vi "胜负对话.vi"(0 "黑子胜？":bool, 1 "白子胜？":bool, 6 "行或列":dbl) -> (14 "x .or. y?":bool, 19 "退出循环？":bool)   [LabVIEW 2018]
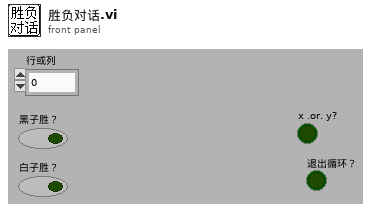
[diagram p1: front panel]
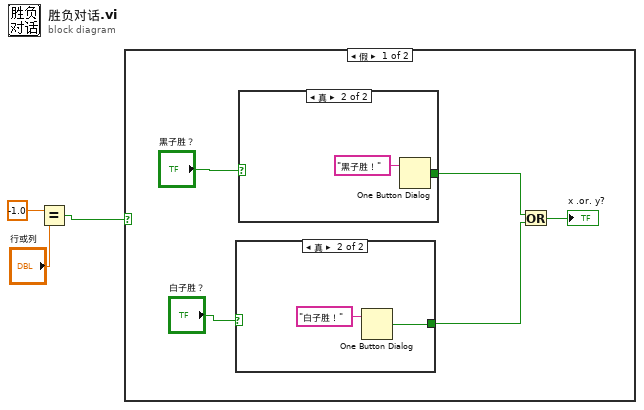
[diagram p0: block diagram]
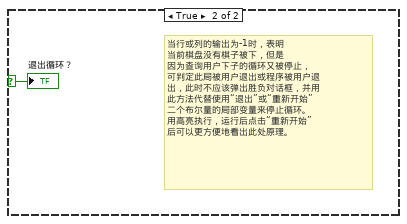
[diagram p4: hidden frame]
diagram:
  n1 = Equal?(x=-1.0, y="行或列") -> (x = y?=w3:bool)
  n2 = case shown="假" w3 {
    selector: w3 -> [_ w13]
    frame False {
      n3 = case shown="真" "白子胜？" {
        tunnel: [_ w9] -> w5
        frame False {
        }
        frame True {
          n4 = One Button Dialog(message="白子胜！") -> (true=w9:bool)  [unwired: 1 in]
        }
      }
      n5 = case shown="真" "黑子胜？" {
        tunnel: [_ w11] -> w6
        frame False {
        }
        frame True {
          n6 = One Button Dialog(message="黑子胜！") -> (true=w11:bool)  [unwired: 1 in]
        }
      }
      n7 = Or(x=w6, y=w5) -> (x .or. y?=→"x .or. y?":bool)
    }
    frame True {
      # "当行或列的输出为-1时，表明\n当前棋盘没有棋子被下，但是\n因为查询用户下子的循环又被停止，\n可判定此局被用户退出或程序被用户退\n出，此时不应该弹出胜负对话框，并用\n此方法代替使用“退出”或“重新开始”\n二个布尔量的局部变量来停止循环。\n用高亮执行，运行后点击“重新开始”\n后可以更方便地看出此处原理。"
      "退出循环？" <- w13
    }
  }
